vi "comm bytes at port.vi"(8 "error in (no error)":errorcluster, 11 "Comm Handle":u64) -> (0 "error out":errorcluster, 2 "bytes at port":u32, 3 "dup Comm Handle":u64)   [LabVIEW 2021, in "lvserial.lvlib"]
doc: "Number of bytes received by the serial provider but not yet read by a ReadFile operation."
uses:
  lvserial.lvlib
  lvserial.dll
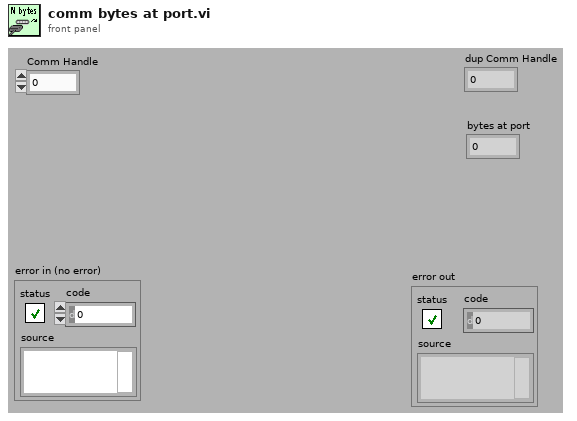
[diagram p1: front panel]
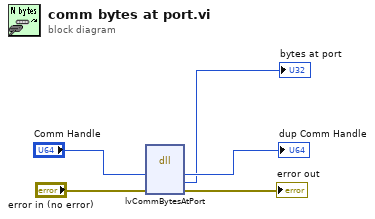
[diagram p0: block diagram]
diagram:
  n1 = dll-call lib="lvserial.dll" fn="lvCommBytesAtPort"("hComm"="Comm Handle", "error"="error in (no error)") -> ("hComm"=→"dup Comm Handle":u64, "puBytesAtPort"=→"bytes at port":u32, "error"=→"error out":errorcluster)  [unwired: 3 in, 4 out]
